vi "Logout.vi"(11 "Authentication Service in":refnum<class "Authentication Service.lvclass">) -> (3 "Authentication Service out":refnum<class "Authentication Service.lvclass">)   [LabVIEW 2026, in "Authentication Service.lvclass"]
uses:
  Authentication Service.lvclass
  Authentication Service.lvclass/Authentication Service.ctl
  Domain/Session/Session.lvclass
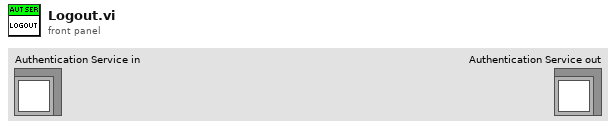
[diagram p1: front panel]
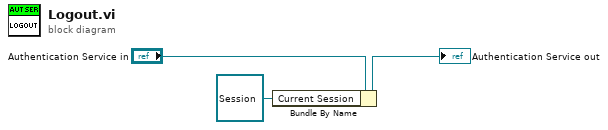
[diagram p0: block diagram]
diagram:
  n1 = Bundle By Name(cluster="Authentication Service in", "Current Session"=refnum<class "Session.lvclass"> refnum) -> (→"Authentication Service out":refnum<class "Authentication Service.lvclass">)
